vi "130725 testScan Alex.vi"() -> ()   [LabVIEW 2013]
uses:
  <vilib>/Utility/file.llb/Write To Spreadsheet File (DBL).vi
panel:
  out "Y2":dbl
  out "X2":dbl
  out "Y1":dbl
  out "X1":dbl
  out "Cryostat Temp 2":dbl format="%.3f"
  out "Probe Temp 2":dbl format="%.3f"
  in  "Tab Control":enum32{"Page 1", "DeltaX vs T", "DeltaY vs T"}(tab)
  in  "Set Point":dbl
  in  "Lock in\nGPIB Address 1":i16
  in  "Save file path":path
  in  "error in (no error)":errorcluster
  in  "Cooling":bool
  in  "LKS\nGPIB Address":i16
  in  "Seconds to sample":dbl
  in  "Lock in\nGPIB Address 2":i16
  out "XY Graph 4":cluster{dbl, dbl}[](graph) caption="XY Graph"
  out "XY Graph 5":cluster{dbl, dbl}[](graph) caption="XY Graph"
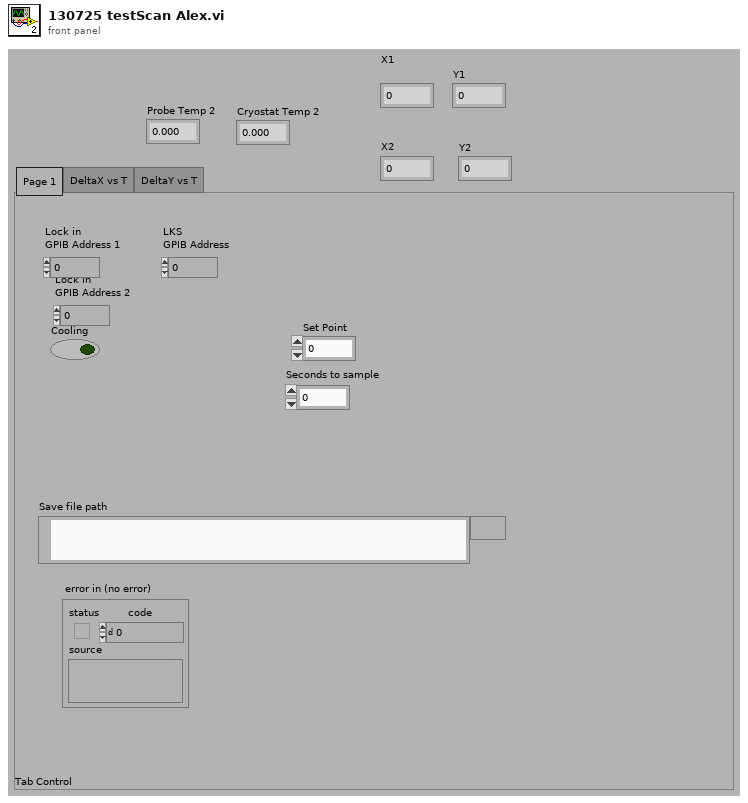
[diagram p1: front panel]
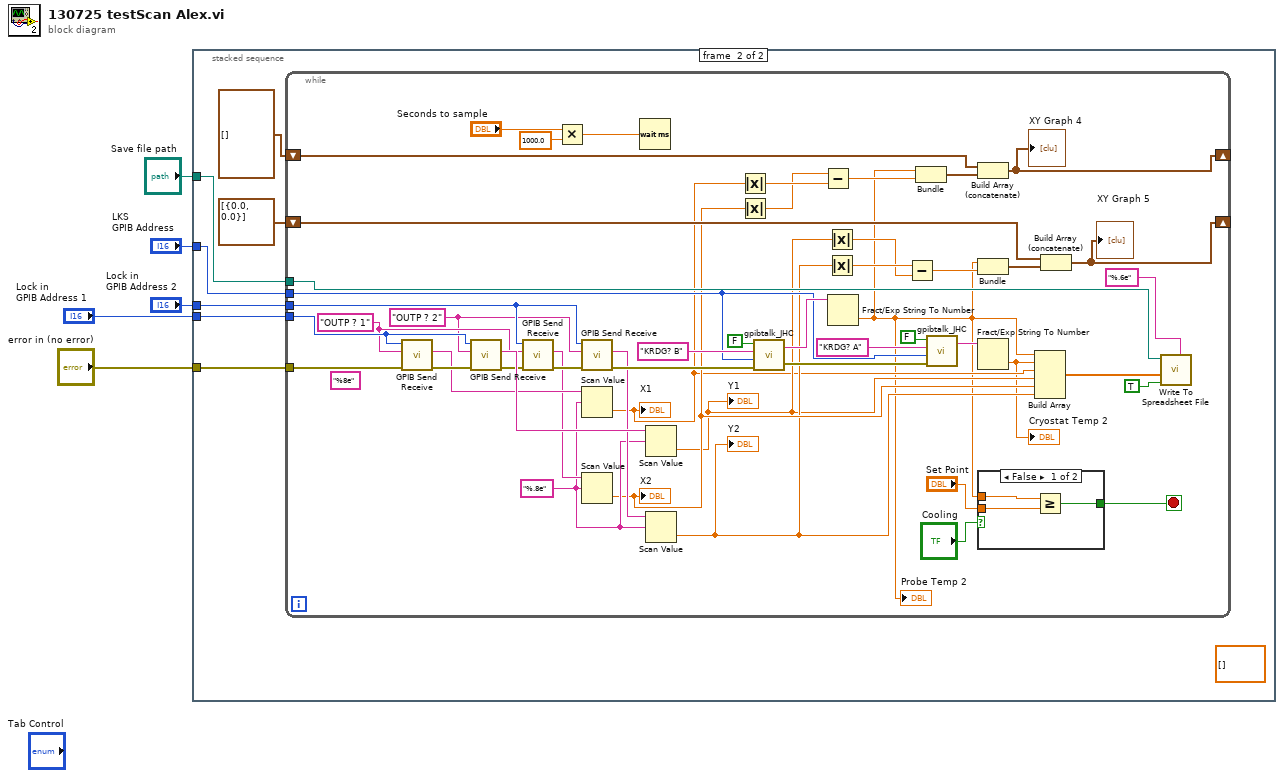
[diagram p0: block diagram]
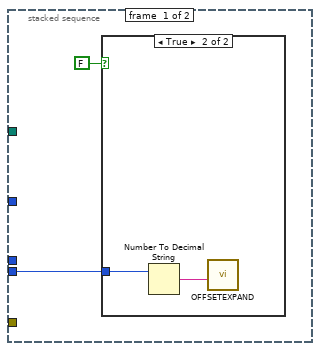
[diagram p2: hidden frame]
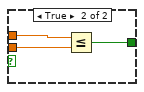
[diagram p4: hidden frame]
diagram:
  n1 = stacked-sequence {
    tunnel: "error in (no error)" -> [_ w15]
    tunnel: "Lock in\nGPIB Address 1" -> [w7 w14]
    tunnel: "Save file path" -> [_ w13]
    tunnel: "LKS\nGPIB Address" -> [_ w12]
    tunnel: "Lock in\nGPIB Address 2" -> [_ w11]
    frame #0 {
      n2 = case shown="True" FALSE {
        tunnel: w7 -> [_ w8]
        frame False {
        }
        frame True {
          n3 = Number To Decimal String(number=w8) -> (decimal integer string=w9:string)  [unwired: 1 in]
          n4 = call "OFFSETEXPAND.vi"("address string"=w9) -> ()  [unwired: 11 in]
        }
      }
    }
    frame #1 {
      (unwired) dbl[][] []
      n5 = while {
        shift-right: [w66] -> _
        shift-left: cluster{dbl, dbl}[] [] -> [w59]
        tunnel: w15 -> [w54]
        tunnel: w14 -> [w55]
        tunnel: w13 -> [w46]
        tunnel: w12 -> [w45]
        tunnel: w11 -> [w38]
        shift-right: [w31] -> _
        shift-left: cluster{dbl, dbl}[] [{0.0, 0.0}] -> [w34]
        stop <- w50 stop-if-true
        (unwired) "%8e" ("format string")
        w27 = "%.8e" ("format string")
        w36 = "OUTP ? 2" ("data string in")
        w37 = "OUTP ? 1" ("data string in")
        n6 = call "GPIB Send Receive.vi"("error in (no error)"=w54, "data string in"=w37, "GPIB Adress"=w55) -> ("error out"=w60:errorcluster, "data string out"=w30:string)  [unwired: 6 in, 1 out]
        n7 = call "GPIB Send Receive.vi"("error in (no error)"=w60, "data string in"=w36, "GPIB Adress"=w55) -> ("error out"=w41:errorcluster, "data string out"=w58:string)  [unwired: 6 in, 1 out]
        n8 = call "GPIB Send Receive.vi"("error in (no error)"=w41, "data string in"=w37, "GPIB Adress"=w38) -> ("error out"=w40:errorcluster, "data string out"=w29:string)  [unwired: 6 in, 1 out]
        n9 = Multiply(x="Seconds to sample", y=1000.0) -> (x*y=w42:dbl)
        n10 = call "GPIB Send Receive.vi"("error in (no error)"=w40, "data string in"=w36, "GPIB Adress"=w38) -> ("error out"=w39:errorcluster, "data string out"=w28:string)  [unwired: 6 in, 1 out]
        n11 = Scan Value(string=w30, format string=w27) -> (value=w19:dbl)  [unwired: 1 in, 1 out]
        "X1" <- w19
        n12 = Scan Value(string=w29, format string=w27) -> (value=w24:dbl)  [unwired: 1 in, 1 out]
        "X2" <- w24
        n13 = Wait (ms)(milliseconds to wait=w42) -> ()  [unwired: 1 out]
        n14 = Scan Value(string=w58, format string=w27) -> (value=w20:dbl)  [unwired: 1 in, 1 out]
        "Y1" <- w20
        n15 = Scan Value(string=w28, format string=w27) -> (value=w21:dbl)  [unwired: 1 in, 1 out]
        "Y2" <- w21
        n16 = Absolute Value(x=w19) -> (abs(x)=w26:dbl)
        n17 = Absolute Value(x=w24) -> (abs(x)=w25:dbl)
        n18 = call "gpibtalk_JHC.vi"("error in"=w39, "milliseconds to wait (10)"=w45, "Send"="KRDG? B", "Inst (F:Temp T:Res)"=FALSE ("Inst (T:Temp F:Res)")) -> ("error out"=w61:errorcluster, "read"=w57:string)
        n19 = Subtract(x=w25, y=w26) -> (x-y=w35:dbl)
        n20 = Absolute Value(x=w20) -> (abs(x)=w22:dbl)
        n21 = Absolute Value(x=w21) -> (abs(x)=w23:dbl)
        n22 = Fract/Exp String To Number(string=w57) -> (number=w18:dbl)  [unwired: 3 in, 1 out]
        "Probe Temp 2" <- w18
        n23 = Subtract(x=w23, y=w22) -> (x-y=w32:dbl)
        n24 = Bundle(w18, w35) -> (w53:cluster{dbl, dbl})  [unwired: 1 in]
        n25 = call "gpibtalk_JHC.vi"("error in"=w61, "milliseconds to wait (10)"=w45, "Send"="KRDG? A", "Inst (F:Temp T:Res)"=FALSE ("Inst (T:Temp F:Res)")) -> ("read"=w56:string)  [unwired: 1 out]
        n26 = Build Array (concatenate)(w59, w53) -> (w66:cluster{dbl, dbl}[])
        "XY Graph 4" <- w66
        n27 = Bundle(w18, w32) -> (w33:cluster{dbl, dbl})  [unwired: 1 in]
        n28 = Fract/Exp String To Number(string=w56) -> (number=w17:dbl)  [unwired: 3 in, 1 out]
        "Cryostat Temp 2" <- w17
        n29 = case shown="False" "Cooling" {
          tunnel: w18 -> [w68 w72]
          tunnel: "Set Point" -> [w69 w71]
          tunnel: [w67 w70] -> w50
          frame False {
            n30 = Greater Or Equal?(x=w68, y=w69) -> (x >= y?=w67:bool)
          }
          frame True {
            n31 = Less Or Equal?(x=w72, y=w71) -> (x <= y?=w70:bool)
          }
        }
        n32 = Build Array(w18, w17, w19, w20, w24, w21) -> (w47:dbl[])
        n33 = Build Array (concatenate)(w34, w33) -> (w31:cluster{dbl, dbl}[])
        "XY Graph 5" <- w31
        n34 = call-poly <vilib>:"Write To Spreadsheet File.vi"("format (%.3f)"="%.6e", "append to file? (new file:F)"=TRUE, "1D data"=w47, "file path (dialog if empty)"=w46) -> ()  [unwired: 4 in, 1 out]
      }
    }
  }
